vi "NR Configure ModAcc.vi"(0 "RFmx Handle In":refnum<k21>, 1 "Selector String":string, 5 "NR ModAcc Configuration":T1={"Measurement Length Unit"=1, "Measurement Offset"=0.0, "Measurement Length"=1.0, "EVM Unit"=0, "Averaging Enabled"=0, "Averaging Count"=10} {"Averaging Enabled" items=["False", "True"]; "EVM Unit" items=["Percentage", "dB"]; "Measurement Length Unit" items=["Slot"=1, "Subframe"=3, "Time"=6]}, 11 "error in (no error)":errorcluster) -> (4 "RFmx Handle Out":refnum<k21>, 15 "error out":errorcluster)   [LabVIEW 2016, in "RFmxNR.lvlib"]
uses:
  RFmxNR.lvlib
  Typedefs/NR ModAcc Configuration.ctl
  <vilib>/RFmx/NR/mx/RFmxNR.llb/RFmxNR Select Measurement (Single).vi
  <resource>/objmgr/RFmxNR.rc
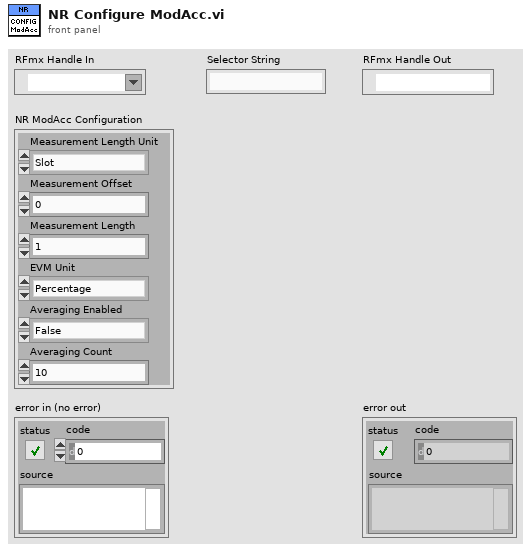
[diagram p1: front panel]
types:
  T1 = typedef "RFmxNR.lvlib/NR ModAcc Configuration.ctl" = cluster{"Measurement Length Unit":i32, "Measurement Offset":dbl, "Measurement Length":dbl, "EVM Unit":i32, "Averaging Enabled":i32, "Averaging Count":i32}
  T2 = enum16{"ModAcc", "SEM", "ACP", "CHP", "OBW", "PVT"}
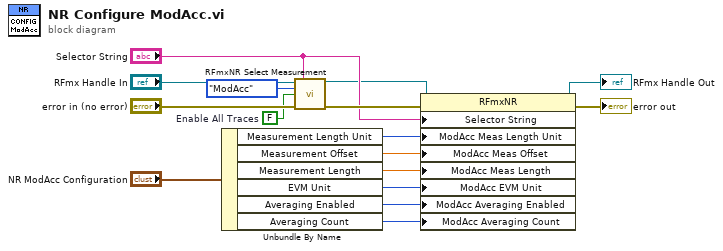
[diagram p0: block diagram]
diagram:
  w1 = FALSE  # Enable All Traces
  n1 = Unbundle By Name("NR ModAcc Configuration") -> ("Measurement Length Unit"=w12:i32, "Measurement Offset"=w11:dbl, "Measurement Length"=w10:dbl, "EVM Unit"=w9:i32, "Averaging Enabled"=w8:i32, "Averaging Count"=w7:i32)
  n2 = call-poly <vilib>:"RFmxNR Select Measurement.vi"("Instrument Handle In"="RFmx Handle In", "Selector String"="Selector String", "Measurement"=T2."ModAcc", "Enable All Traces"=w1, "error in (no error)"="error in (no error)") -> ("Instrument Handle Out"=w4:refnum<k21>, "error out"=w14:errorcluster)  [unwired: 9 in]
  n3 = property class="RFmxNR"(reference=w4, error in=w14, "Selector String"="Selector String", "ModAcc Meas Length Unit"=w12, "ModAcc Meas Offset"=w11, "ModAcc Meas Length"=w10, "ModAcc EVM Unit"=w9, "ModAcc Averaging Enabled"=w8, "ModAcc Averaging Count"=w7) -> (reference out=→"RFmx Handle Out":refnum<k21>, error out=→"error out":errorcluster)
